vi "Trim Whitespace (String)__ogtk.vi"(5 "Remove (leading and trailing)":enum16{"leading", "trailing", "both"}(ring)=enum."both", 6 "String in":string) -> (1 "String out":string)   [LabVIEW 2012]
doc: "Removes leading and/or trailing whitespace from a string.\nWhitespace is defined as any of the following characters (where values are in the format: dec, hex, string):\n <b>tab</b> = 9, 0x09, \\t\n <b>newline</b> = 10, 0x0A, \\n\n <b>vertical tab</b> = 11, 0x0B, \\0B\n <b>form feed</b> = 12, 0x0C, \\f\n <b>carriage return</b> = 13, 0x0D, \\r \n <b>space</b> = 32, 0x20, \\s\n\nThis VI 's execution is set to <b>subroutine</b>\nThis VI is <b>reentrant</b>"
panel:
  # "Trim Whitespace (String) 1.vi\n\nRemoves leading and/or trailing whitespace from a string.\n\nPlease visit http://www.OpenG.org to learn about the\nOpen Source LabVIEW software movement.\n\nNOTICE -- YOU MUST LEAVE THIS NOTICE IN PLACE.  PER THE TERMS OF THE LICENSE BELOW, YOU MAY SUBLICENSE THIS SOFTWARE \nIN ANY WAY THAT DOES NOT CONFLICT WITH THIS LICENSE.\n\n### BSD License (http://www.opensource.org/licenses/bsd-license.php) Begin ###\n\nCopyright (c) 2002-2006, Jim Kring <jim@jimkring.com>\nCopyright (c) 2002, Cal-Bay Systems, Inc. <info@calbay.com>\nCopyright (c) 2011,  Shaun Rumbell <shaunr@labview-tools.com> \nCopyright (c) 2011,  Darin.K <darin@alum.mit.edu>\nCopyright (c) 2011, Jonathon Green <jg@jgcode.net>\n\nAll rights reserved.\n\nRedistribution and use in source and binary forms, with or without modification, are permitted provided that the following conditions are met:\n\n    * Redistributions of source code must retain the above copyright notice, this list of conditions and the following disclaimer.\n    * Redistributions in binary form must reproduce the above copyright notice, this list of conditions and the following disclaimer in the \n       documentation and/or other materials provided with the distribution.\n    * Neither the name of SciWare, James Kring, Inc., nor the names of its contributors may be used to endorse or promote products derived \n       from this software without specific prior written permission.\n\nTHIS SOFTWARE IS PROVIDED BY THE COPYRIGHT HOLDERS AND CONTRIBUTORS \"AS IS\" AND ANY EXPRESS OR IMPLIED WARRANTIES, \nINCLUDING, BUT NOT LIMITED TO, THE IMPLIED WARRANTIES OF MERCHANTABILITY AND FITNESS FOR A PARTICULAR PURPOSE ARE \nDISCLAIMED. IN NO EVENT SHALL THE COPYRIGHT OWNER OR CONTRIBUTORS BE LIABLE FOR ANY DIRECT, INDIRECT, INCIDENTAL,\n SPECIAL, EXEMPLARY, OR CONSEQUENTIAL DAMAGES (INCLUDING, BUT NOT LIMITED TO, PROCUREMENT OF SUBSTITUTE GOODS OR \nSERVICES; LOSS OF USE, DATA, OR PROFITS; OR BUSINESS INTERRUPTION) HOWEVER CAUSED AND ON ANY THEORY OF LIABILITY, \nWHETHER IN CONTRACT, STRICT LIABILITY, OR TORT (INCLUDING NEGLIGENCE OR OTHERWISE) ARISING IN ANY WAY OUT OF THE USE \nOF THIS SOFTWARE, EVEN IF ADVISED OF THE POSSIBILITY OF SUCH DAMAGE.\n\n### BSD License End ###"
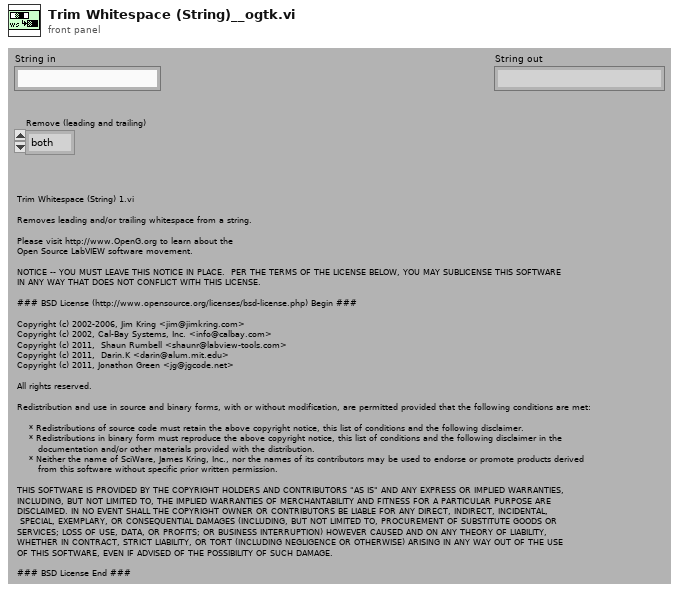
[diagram p1: front panel]
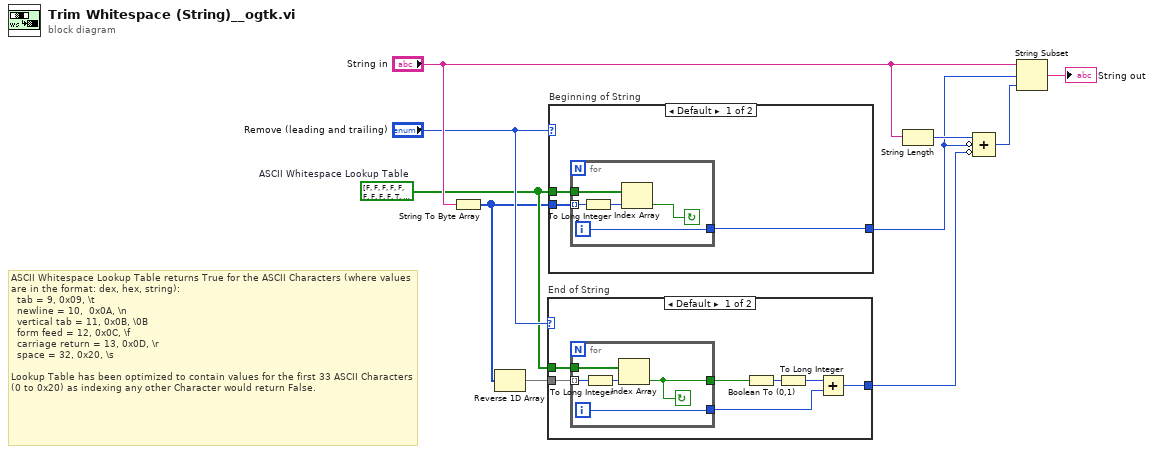
[diagram p0: block diagram]
diagram:
  w2 = bool[] [FALSE, FALSE, FALSE, FALSE, FALSE, FALSE, FALSE, FALSE, FALSE, TRUE, TRUE, TRUE, TRUE, TRUE, FALSE, FALSE, FALSE, FALSE, FALSE, FALSE, FALSE, FALSE, FALSE, FALSE, FALSE, FALSE, FALSE, FALSE, FALSE, FALSE, FALSE, FALSE, TRUE]  # ASCII Whitespace Lookup Table
  # "ASCII Whitespace Lookup Table returns True for the ASCII Characters (where values are in the format: dex, hex, string):\n  tab = 9, 0x09, \\t\n  newline = 10,  0x0A, \\n\n  vertical tab = 11, 0x0B, \\0B\n  form feed = 12, 0x0C, \\f\n  carriage return = 13, 0x0D, \\r \n  space = 32, 0x20, \\s\n\nLookup Table has been optimized to contain values for the first 33 ASCII Characters (0 to 0x20) as indexing any other Character would return False."
  n1 = String To Byte Array(string="String in") -> (unsigned byte array=w1:u8[])
  n2 = Reverse 1D Array(array=w1) -> (reversed array=w9:u8[])
  n3 = case "End of String" shown="Default" "Remove (leading and trailing)" {
    tunnel: w9 -> [w17 _]
    tunnel: [w15 _] -> w3
    tunnel: w2 -> [w12 _]
    frame Default {
      n4 = for {
        tunnel: w17 -> [w19] mode=indexing
        tunnel: [w22] -> w16
        tunnel: [w20] -> w11
        tunnel: w12 -> [w21]
        i -> [w22]
        stop <- w20 continue-if-true
        n5 = To Long Integer(number=w19) -> (32bit integer=w18:i32)
        n6 = Index Array(array=w21, index=w18) -> (element=w20:bool)
      }
      n7 = Boolean To (0,1)(Boolean=w11) -> (0, 1=w14:i16)
      n8 = To Long Integer(number=w14) -> (32bit integer=w13:i32)
      n9 = Add(x=w13, y=w16) -> (x+y=w15:i32)
    }
    frame "leading" {
    }
  }
  n10 = case "Beginning of String" shown="Default" "Remove (leading and trailing)" {
    tunnel: w1 -> [w25 _]
    tunnel: [w24 _] -> w4
    tunnel: w2 -> [w23 _]
    frame Default {
      n11 = for {
        tunnel: w25 -> [w27] mode=indexing
        tunnel: [w30] -> w24
        tunnel: w23 -> [w29]
        i -> [w30]
        stop <- w28 continue-if-true
        n12 = To Long Integer(number=w27) -> (32bit integer=w26:i32)
        n13 = Index Array(array=w29, index=w26) -> (element=w28:bool)
      }
    }
    frame "trailing" {
    }
  }
  n14 = String Length(string="String in") -> (length=w7:i32)
  n15 = Compound Arithmetic op=ADD(w7, invert w4, invert w3) -> (w8:i32)
  n16 = String Subset(string="String in", offset (0)=w4, length (rest)=w8) -> (substring=→"String out":string)
